vi "Source_Image name format specifier.vi"() -> (4 "Z-Stack Image name format specifier":string, 5 "Red channel name":string, 7 "Green channel name":string)   [LabVIEW 2017]
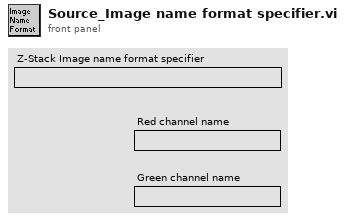
[diagram p1: front panel]
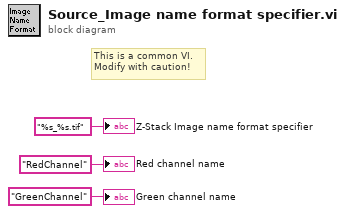
[diagram p0: block diagram]
diagram:
  # "This is a common VI.\nModify with caution!"
  "Z-Stack Image name format specifier" <- "%s_%s.tif" ("format string")
  "Red channel name" <- "RedChannel" ("String")
  "Green channel name" <- "GreenChannel" ("String")
